vi "7-zip tester.vi"   [LabVIEW 2020, in "7-zip Wrapper.lvclass"]
uses:
  7-zip Wrapper.lvclass
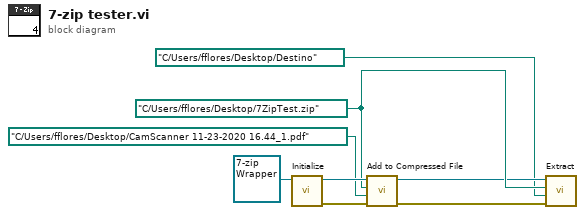
[diagram p0: block diagram]
diagram:
  w4 = path "C:/Users/fflores/Desktop/7ZipTest.zip" ("Compressed File Path")
  n1 = call-dynamic "Initialize.vi"("7-zip Wrapper in"=refnum<class "7-zip Wrapper.lvclass"> refnum) -> ("error out"=w7:errorcluster, "7-zip Wrapper out"=w8:refnum<class "7-zip Wrapper.lvclass">)  [unwired: 9 in]
  n2 = call "Add to Compressed File.vi"("error in (no error)"=w7, "File or Folder to be compressed"=path "C:/Users/fflores/Desktop/CamScanner 11-23-2020 16.44_1.pdf", "Compressed File Path"=w4, "7-zip Wrapper in"=w8) -> ("error out"=w2:errorcluster, "7-zip Wrapper out"=w3:refnum<class "7-zip Wrapper.lvclass">)  [unwired: 6 in]
  n3 = call "Extract.vi"("error in (no error)"=w2, "Destination Folder"=path "C:/Users/fflores/Desktop/Destino" ("Compressed File Path"), "Compressed File Path"=w4, "7-zip Wrapper in"=w3) -> ()  [unwired: 6 in, 2 out]
